vi "Sort Node Terminals.vi"(8 "error in (no error)":errorcluster, 11 "Terms in":refnum<vi>[](array[refnum])) -> (0 "error out":errorcluster, 2 "Top Right":refnum<vi>, 3 "Top Left":refnum<vi>, 4 "Error Left":refnum<vi>, 6 "Error Right":refnum<vi>)   [LabVIEW 2016]
uses:
  <resource>/dialog/QuickDrop/plugins/_WireMultipleSupport/Connector Pane Position.ctl
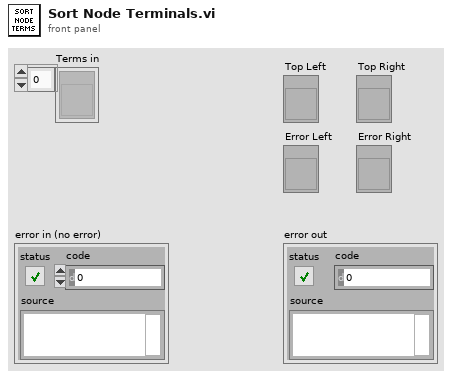
[diagram p1: front panel]
types:
  T1 = typedef "Connector Pane Position.ctl" = enum16{"left", "right"}
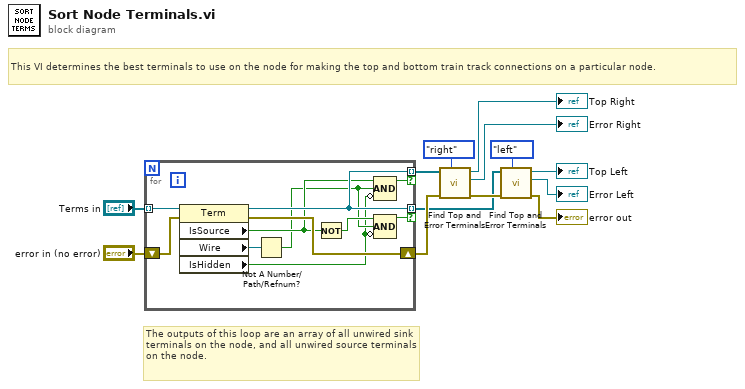
[diagram p0: block diagram]
diagram:
  # "This VI determines the best terminals to use on the node for making the top and bottom train track connections on a particular node."
  # "The outputs of this loop are an array of all unwired sink terminals on the node, and all unwired source terminals on the node."
  n1 = for {
    shift-right: [w22] -> w11
    shift-left: "error in (no error)" -> [w23]
    tunnel: "Terms in" -> [w24] mode=indexing
    tunnel: [w21] -> w1 mode=indexing if=w17
    tunnel: [w21] -> w10 mode=indexing if=w18
    n2 = property class="Term"(reference=w24, error in=w23) -> (reference out=w21:refnum<vi>, error out=w22:errorcluster, "IsSource"=w20:bool, "Wire"=w19:refnum<vi>, "IsHidden"=w14:bool)
    n3 = Not A Number/Path/Refnum?(number/path/refnum=w19) -> (NaN/Path/Refnum?=w15:bool)
    n4 = Not(x=w20) -> (.not. x?=w16:bool)
    n5 = Compound Arithmetic op=AND(w20, w15, invert w14) -> (w18:bool)
    n6 = Compound Arithmetic op=AND(w16, w15, invert w14) -> (w17:bool)
  }
  n7 = call <resource>:"Find Top and Error Terminals.vi"("Position"=Connector_Pane_Position."right", "error in (no error)"=w11, "Array"=w10) -> ("error out"=w6:errorcluster, "Error out"=→"Error Right":refnum<vi>, "Top out"=→"Top Right":refnum<vi>)  [unwired: 6 in]
  n8 = call <resource>:"Find Top and Error Terminals.vi"("Position"=Connector_Pane_Position."left", "error in (no error)"=w6, "Array"=w1) -> ("error out"=→"error out":errorcluster, "Error out"=→"Error Left":refnum<vi>, "Top out"=→"Top Left":refnum<vi>)  [unwired: 6 in]
